vi "Test_RequestSynchronousDatum_DoubleX_ValuePublished_ValueReceived.vi"(8 "error in (no error)":errorcluster, 11 "TestCase in":refnum<class "TestRequestSynchronousData.lvclass">) -> (0 "error out":errorcluster, 3 "TestCase out":refnum<class "TestRequestSynchronousData.lvclass">)   [LabVIEW 2020, in "TestRequestSynchronousData.lvclass"]
uses:
  TestRequestSynchronousData.lvclass
  TestRequestSynchronousData.lvclass/TestRequestSynchronousData.ctl
  24bf8875-c008-4f22-9bfa-88e42476d167.vi
  Source/IModel/IModel/IModel.lvclass
  Doubles/RootModelPublishesDoubleFloatX/RootModelPublishesDoubleFloatX.lvclass
  C:/Git/mva-core/Source/RootModel/RootModel/RootModel.lvclass
  C:/Git/mva-core/Source/IModel/IModel/IModel.lvclass
  C:/Git/mva-core/Source/IObserver/IObserver/IObserver.lvclass
  C:/Program Files (x86)/National Instruments/LabVIEW 2020/vi.lib/ActorFramework/Actor/Actor.lvclass
  C:/Git/mva-core/Test/Doubles/RootModelPublishesDoubleFloatX/RootModelPublishesDoubleFloatX.lvclass
  <vilib>/ActorFramework/Actor/Actor.lvclass
  Source/Mediator/Mediator/Mediator.lvclass
  <vilib>/ActorFramework/Stop Msg/Stop Msg.lvclass
  modules/composed-event-logger/Source/String Control Sink/String Control Sink.lvclass
  f7bee35d-b044-4098-91af-55574313c386.vi
  modules/composed-event-logger/Source/Composed Log/LoggerReference/LoggerReference.lvclass
  11850773-0e08-463b-84b0-7f64b956e994.vi
  Doubles/ModelSynchronouslyRequestsDoubleFloat/ModelSynchronouslyRequestsDoubleFloat.lvclass
  C:/Git/mva-core/Test/Doubles/ModelSynchronouslyRequestsDoubleFloat/ModelSynchronouslyRequestsDoubleFloat.lvclass
panel:
  out "Request Result":T1
  out "Log":string
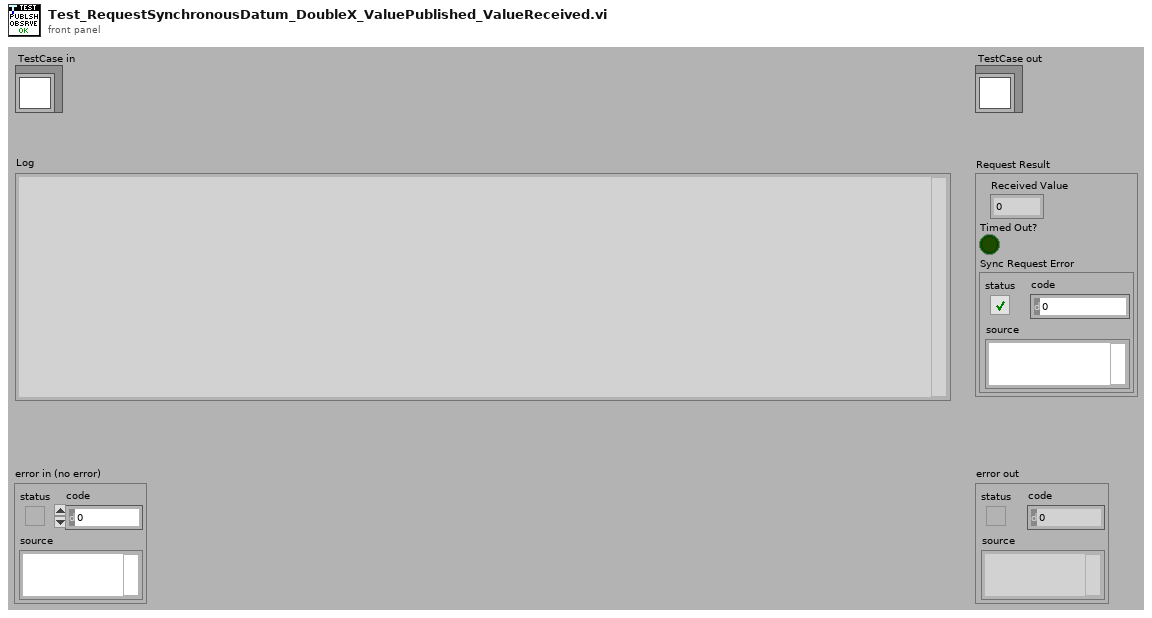
[diagram p1: front panel]
types:
  T1 = cluster{"Received Value":dbl, "Timed Out?":bool, "Sync Request Error":errorcluster}
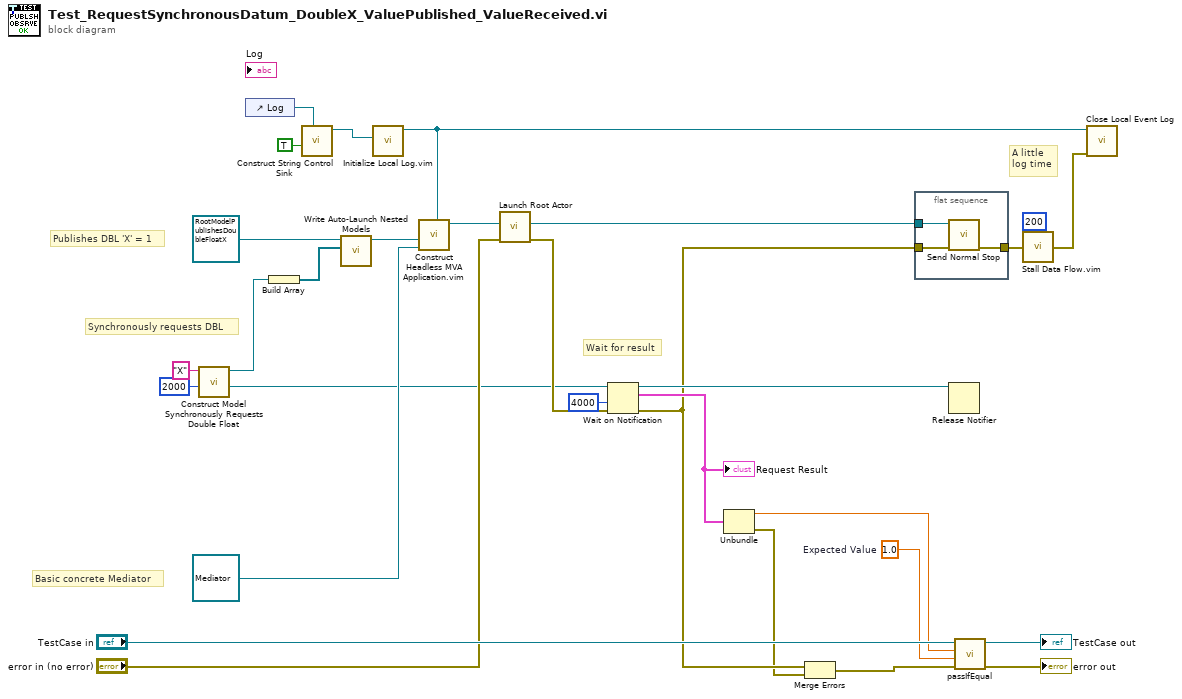
[diagram p0: block diagram]
diagram:
  w19 = 1.0  # Expected Value
  # "A little\nlog time"
  # "Wait for result"
  # "Basic concrete Mediator"
  # "Synchronously requests DBL"
  # "Publishes DBL 'X' = 1"
  n1 = call "Construct Model Synchronously Requests Double Float.vi"("DBL Request Timeout (2000)"=2000, "DBL Name"="X") -> ("Result Notifier"=w16:refnum<notifier>, "ModelSynchronouslyRequestsDoubleFloat Out"=w8:refnum<class "ModelSynchronouslyRequestsDoubleFloat.lvclass">)  [unwired: 8 in]
  n2 = control-ref of="Log"() -> (w15:refnum<vi>)
  n3 = Build Array(w8) -> (w26:refnum<class "ModelSynchronouslyRequestsDoubleFloat.lvclass">[])
  n4 = call "Construct String Control Sink.vi"("Str Refnum"=w15, "AutoScroll?(F)"=TRUE) -> ("String Control Sink out"=w14:refnum<class "String Control Sink.lvclass">)  [unwired: 9 in]
  n5 = call "Write Auto-Launch Nested Models.vi"("Auto-Launch Nested Models"=w26, "IModel In"=refnum<class "RootModelPublishesDoubleFloatX.lvclass"> refnum ("RootModelPublishesDoubleFloatX.lvclass")) -> ("IModel Out"=w25:refnum<class "RootModelPublishesDoubleFloatX.lvclass">)  [unwired: 9 in]
  n6 = call "Initialize Local Log.vim"("Startup Sink(s)"=w14) -> ("Log Instance Reference"=w12:refnum<class "LoggerReference.lvclass">)  [unwired: 8 in, 2 out]
  n7 = call "Construct Headless MVA Application.vim"("Parent Log Reference"=w12, "Mediator Type"=refnum<class "Mediator.lvclass"> refnum ("Mediator.lvlib:Mediator.lvclass"), "RootModel in"=w25) -> ("RootModel out"=w24:refnum<class "RootModelPublishesDoubleFloatX.lvclass">)  [unwired: 8 in]
  n8 = call <vilib>:"Launch Root Actor.vi"("error in (no error)"="error in (no error)", "Actor"=w24) -> ("error out"=w20:errorcluster, "Actor's Enqueuer"=w18:refnum<class "Message Enqueuer.lvclass">)  [unwired: 8 in]
  n9 = Wait on Notification(notifier=w16, timeout in ms (-1)=4000, error in (no error)=w20) -> (notifier out=w23:refnum<notifier>, notification=w4:T1, error out=w3:errorcluster)  [unwired: 1 in, 1 out]
  "Request Result" <- w4
  n10 = Unbundle(w4) -> ("Received Value"=w5:dbl, "Sync Request Error"=w1:errorcluster)  [unwired: 1 out]
  n11 = Merge Errors(w3, w1) -> (w2:errorcluster)
  n12 = flat-sequence {
    tunnel: w18 -> [w33]
    tunnel: [w32] -> w11
    tunnel: w3 -> [w31]
    frame #0 {
      n13 = call <vilib>:"Send Normal Stop.vi"("error in (no error)"=w31, "Message Enqueuer"=w33) -> ("error out"=w32:errorcluster)  [unwired: 9 in]
    }
  }
  n14 = Release Notifier(notifier=w23) -> ()  [unwired: 2 in, 3 out]
  n15 = call-dynamic "passIfEqual.vi"("error in (no error)"=w2, "y"=w19, "x"=w5, "TestCase in"="TestCase in") -> ("error out"=→"error out":errorcluster, "TestCase out"=→"TestCase out":refnum<class "TestRequestSynchronousData.lvclass">)  [unwired: 6 in]
  n16 = call "Stall Data Flow.vim"("value in"=w11, "milliseconds to wait"=u32 200) -> ("value out"=w10:errorcluster)  [unwired: 1 out]
  n17 = call "Close Local Event Log.vi"("error in (no error)"=w10, "Log Instance"=w12) -> ()  [unwired: 9 in, 1 out]
